vi "Warn.vi"(6 "sound?":bool, 8 "NwarnIN":bool, 9 "HwarnIN":bool, 10 "warncontN":T1={"alarmliqN"=90.0, "warn?N"=FALSE, "lessthan?N"=FALSE}, 11 "warncontHe":T2={"alarmliqHe"=85.0, "warn?He"=FALSE, "lessthan?He"=FALSE}) -> (2 "warnNOUT":T1={"alarmliqN"=90.0, "warn?N"=FALSE, "lessthan?N"=FALSE}, 3 "warnHeOUT":T2={"alarmliqHe"=85.0, "warn?He"=FALSE, "lessthan?He"=FALSE})   [LabVIEW 2009, in "Magnet.lvclass"]
uses:
  Magnet.lvclass
  Global/Sound Files.vi
panel:
  in  "turnoff":bool
  out "Nwarn":bool caption="LN"
  out "Hwarn":bool caption="LHe"
  in  "exit":bool
  out "disp":string
  out "warn2":bool
  out "warn1":bool
  # "Off"
  # "On"
  # "Greater"
  # "Less"
  # "Off"
  # "On"
  # "Greater"
  # "Less"
  # "Off"
  # "On"
  # "Greater"
  # "Less"
  # "Off"
  # "On"
  # "Greater"
  # "Less"
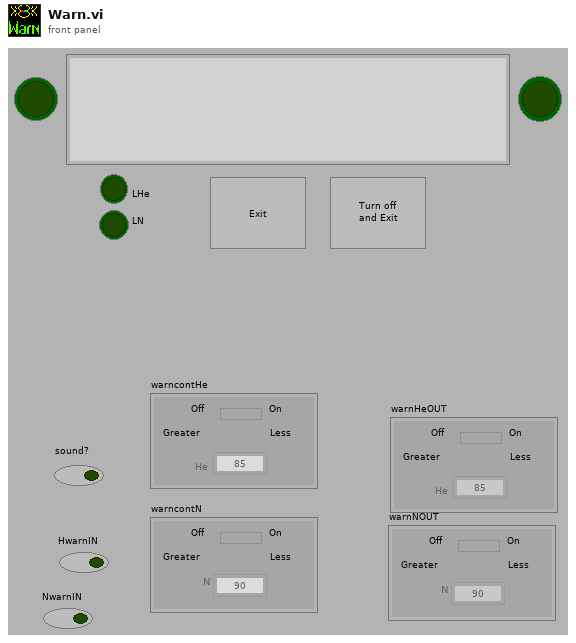
[diagram p1: front panel]
types:
  T1 = cluster{"alarmliqN":dbl, "warn?N":bool, "lessthan?N":bool}
  T2 = cluster{"alarmliqHe":dbl, "warn?He":bool, "lessthan?He":bool}
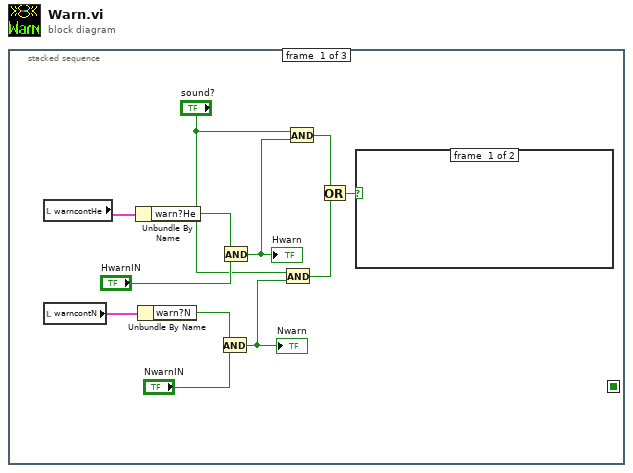
[diagram p0: block diagram]
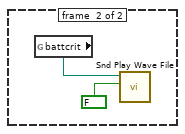
[diagram p2: hidden frame]
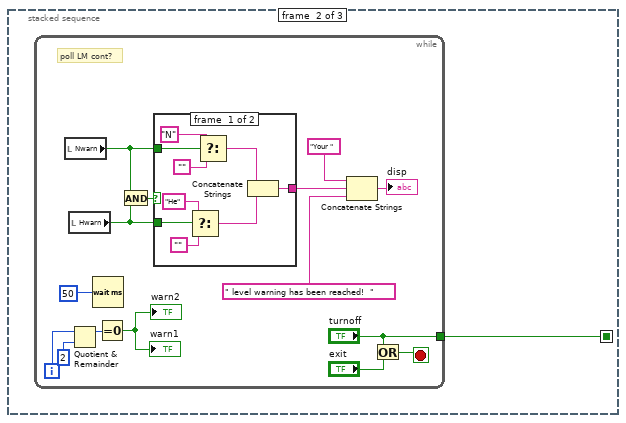
[diagram p3: hidden frame]
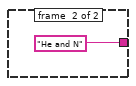
[diagram p4: hidden frame]
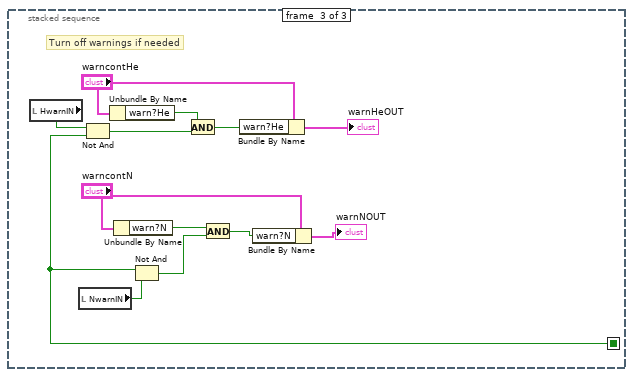
[diagram p5: hidden frame]
diagram:
  n1 = stacked-sequence {
    seq-local: [_ w15 _] -> [_ _ w43]
    frame #0 {
      n2 = local read "warncontHe"() -> (w12:T2)
      n3 = local read "warncontN"() -> (w8:T1)
      n4 = Unbundle By Name(w12) -> ("warn?He"=w11:bool)
      n5 = Unbundle By Name(w8) -> ("warn?N"=w9:bool)
      n6 = And(x=w9, y="NwarnIN") -> (x .and. y?=w5:bool)
      "Nwarn" <- w5
      n7 = And(x=w11, y="HwarnIN") -> (x .and. y?=w6:bool)
      "Hwarn" <- w6
      n8 = And(x="sound?", y=w5) -> (x .and. y?=w2:bool)
      n9 = And(x="sound?", y=w6) -> (x .and. y?=w3:bool)
      n10 = Or(x=w3, y=w2) -> (x .or. y?=w1:bool)
      n11 = case shown="True" w1 {
        frame #0 {
        }
        frame #1 {
          n12 = global read "Sound Files.vi" "battcrit"() -> (w13:path)
          n13 = call <vilib>:"Snd Play Wave File.vi"("wait until finish (T)"=FALSE, "wave file path"=w13) -> ()  [unwired: 1 in, 9 out]
        }
      }
    }
    frame #1 {
      n14 = while {
        tunnel: ["turnoff"] -> w15
        i -> [w30]
        stop <- w17 stop-if-true
        # "poll LM cont?"
        n15 = local read "Nwarn"() -> (w24:bool)
        n16 = local read "Hwarn"() -> (w23:bool)
        n17 = Quotient & Remainder(x=w30, y=2) -> (x-y*floor(x/y)=w29:i32)  [unwired: 1 out]
        n18 = Wait (ms)(milliseconds to wait=50) -> ()  [unwired: 1 out]
        n19 = Equal To 0?(x=w29) -> (x = 0?=→"warn1" →"warn2":bool)
        n20 = And(x=w24, y=w23) -> (x .and. y?=w25:bool)
        n21 = case shown="False" w25 {
          tunnel: w24 -> [w39 _]
          tunnel: w23 -> [w38 _]
          tunnel: [w31 "He and N"] -> w22
          frame #0 {
            n22 = Select(t="He", s=w38, f="") -> (s? t:f=w37:string)
            n23 = Select(t="N", s=w39, f="") -> (s? t:f=w36:string)
            n24 = Concatenate Strings(w36, w37) -> (w31:string)
          }
          frame #1 {
          }
        }
        n25 = Concatenate Strings("Your ", w22, " level warning has been reached!  ") -> (→"disp":string)
        n26 = Or(x="turnoff", y="exit") -> (x .or. y?=w17:bool)
      }
    }
    frame #2 {
      # "Turn off warnings if needed"
      n27 = local read "HwarnIN"() -> (w41:bool)
      n28 = local read "NwarnIN"() -> (w44:bool)
      n29 = Not And(1:w43, 2:w41) -> (0:w47:bool)
      n30 = Unbundle By Name("warncontHe") -> ("warn?He"=w49:bool)
      n31 = Unbundle By Name("warncontN") -> ("warn?N"=w46:bool)
      n32 = Not And(1:w44, 2:w43) -> (0:w42:bool)
      n33 = And(x=w49, y=w47) -> (x .and. y?=w48:bool)
      n34 = And(x=w46, y=w42) -> (x .and. y?=w45:bool)
      n35 = Bundle By Name(cluster="warncontHe", "warn?He"=w48) -> (→"warnHeOUT":T2)
      n36 = Bundle By Name(cluster="warncontN", "warn?N"=w45) -> (→"warnNOUT":T1)
    }
  }
